vi "Logic for Default Case Multiple.vi"(11 "error in (no error)":errorcluster) -> (15 "error out":errorcluster)   [LabVIEW 2021, in "Migrator.lvlib"]
uses:
  Migrator.lvlib
  <vilib>/Utility/traverseref.llb/TRef TravTarget.ctl
  <vilib>/Utility/traverseref.llb/VI Scripting - Traverse.lvlib
  Migrator Reusables/Migrator Reusables.lvlib
  Path Functions/Path Functions.lvlib
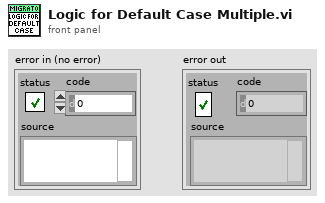
[diagram p1: front panel]
types:
  T1 = typedef "TRef TravTarget.ctl" = enum16{"FP", "BD", "Other"}
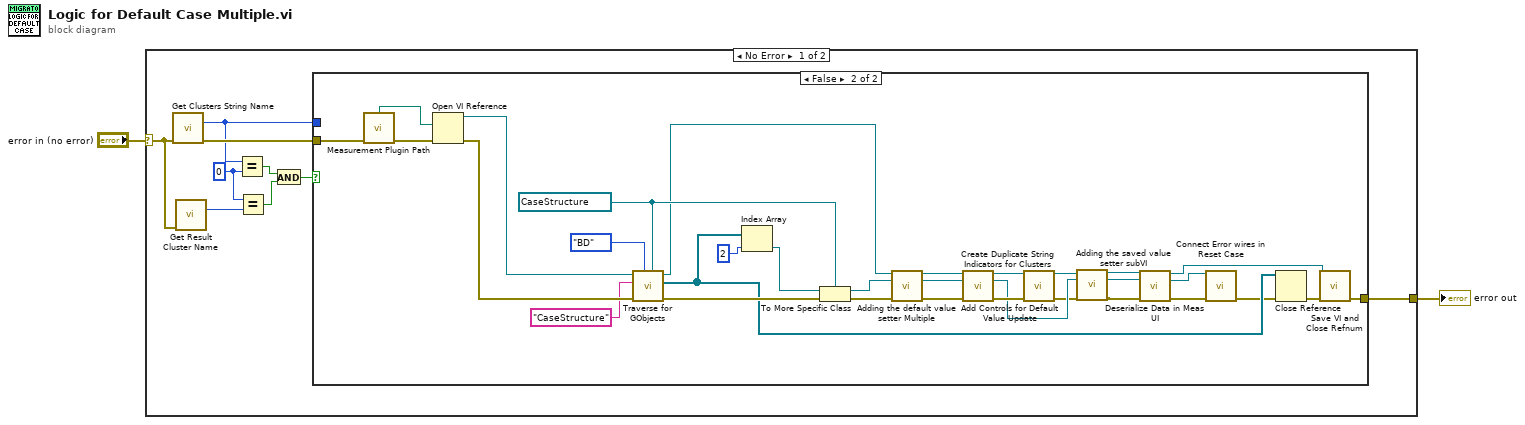
[diagram p0: block diagram]
diagram:
  n1 = case shown="No Error" "error in (no error)" {
    selector: "error in (no error)" -> [w10 w45]
    tunnel: [w11 w45] -> w2
    frame No Error {
      w7 = 0 ("y")
      n2 = call "Get Clusters String Name.vi"("error in (no error)"=w10) -> ("Array Size"=w8:i32, "error out"=w9:errorcluster)  [unwired: 12 in, 1 out]
      n3 = call "Get Result Cluster Name.vi"("error in (no error)"=w10) -> ("Array Size"=w6:i32)  [unwired: 12 in, 2 out]
      n4 = Equal?(x=w8, y=w7) -> (x = y?=w5:bool)
      n5 = Equal?(x=w7, y=w6) -> (x = y?=w4:bool)
      n6 = And(x=w5, y=w4) -> (x .and. y?=w3:bool)
      n7 = case shown="False" w3 {
        tunnel: [w12 w39] -> w11
        tunnel: w9 -> [w12 w19]
        tunnel: w8 -> [_ _]
        frame True {
        }
        frame False {
          w41 = refnum<vi> refnum ("Other Refnum")
          n8 = call "Measurement Plugin Path.vi"("error in (no error)"=w19) -> ("Measurement UI"=w21:path, "error out"=w20:errorcluster)  [unwired: 2 in, 11 out]
          n9 = Open VI Reference(vi path=w21, error in (no error)=w20) -> (vi reference=w35:refnum<vi>, error out=w44:errorcluster)  [unwired: 4 in]
          n10 = call <vilib>:"Traverse for GObjects.vi"("Other Refnum"=w41, "Traverse Target"=TRef_TravTarget."BD", "error in (no error)"=w44, "Class Name"="CaseStructure", "VI Refnum"=w35) -> ("error out"=w40:errorcluster, "References"=w28:refnum<vi>[], "dup VI Refnum"=w18:refnum<vi>)  [unwired: 3 in, 1 out]
          n11 = Index Array(array=w28, index=2) -> (element=w37:refnum<vi>)
          n12 = To More Specific Class(target class=w41, reference=w37, error in=w40) -> (specific class reference=w17:refnum<vi>, error out=w16:errorcluster)
          n13 = call "Adding the default value setter Multiple.vi"("VI in"=w18, "Case Sel Refnum"=w17, "error in (no error)"=w16) -> ("VI Out"=w14:refnum<vi>, "Case Sel Refnum Out"=w13:refnum<vi>, "error out"=w15:errorcluster)  [unwired: 10 in]
          n14 = call "Add Controls for Default Value Update.vi"("VI Refnum"=w14, "Case Sel Refnum"=w13, "error in (no error)"=w15) -> ("VI Refnum Out"=w34:refnum<vi>, "Case Sel Refnum Out"=w32:refnum<vi>, "error out"=w36:errorcluster)  [unwired: 10 in]
          n15 = call "Create Duplicate String Indicators for Clusters.vi"("UI VI Ref"=w34, "error in (no error)"=w36) -> ("UI VI Ref Out"=w33:refnum<vi>, "error out"=w25:errorcluster)  [unwired: 12 in]
          n16 = call "Adding the saved value setter subVI.vi"("VI in"=w33, "Case Sel Refnum"=w32, "error in (no error)"=w25) -> ("VI Out"=w31:refnum<vi>, "Case Sel Refnum Out"=w30:refnum<vi>, "error out"=w26:errorcluster)  [unwired: 10 in]
          n17 = call "Deserialize Data in Meas UI.vi"("VI Refnum"=w31, "Case Sel Refnum"=w30, "error in (no error)"=w26) -> ("VI Refnum Out"=w29:refnum<vi>, "Case Sel Refnum Out"=w24:refnum<vi>, "error out"=w22:errorcluster)  [unwired: 10 in]
          n18 = call "Connect Error wires in Reset Case.vi"("Case Sel Refnum"=w24, "error in (no error)"=w22) -> ("error out"=w23:errorcluster)  [unwired: 12 in, 1 out]
          n19 = Close Reference(reference=w28, error in (no error)=w23) -> (error out=w27:errorcluster)
          n20 = call "Save VI and Close Refnum.vi"("VI Refnum"=w29, "error in"=w27) -> ("error out"=w39:errorcluster)  [unwired: 13 in]
        }
      }
    }
    frame Error {
    }
  }
  "error out" <- w2
